vi "Postprocessing_utility_RA_molecularLine_fileSum.vi"() -> ()   [LabVIEW 2016]
doc: "VI for maser line post-processing"
uses:
  <vilib>/Utility/config.llb/Read Key (Double).vi
  <vilib>/Utility/file.llb/Read Delimited Spreadsheet (DBL).vi
  <vilib>/Utility/file.llb/Write Delimited Spreadsheet (DBL).vi
  <vilib>/Analysis/6fits.llb/1D B-Spline Fit.vi
  <vilib>/Utility/config.llb/NI_LVConfig.lvlib
  <vilib>/Analysis/NI_AALPro.lvlib
panel:
  in  "TabControl":enum32{"Averaging", "Jy&Speed plot"}(tab)
  in  "Frequency_MHz":dbl(knob)=969.0 caption="Frequency, MHz" min=70.0 max=6000.0 scale=70.0..6000.0 scale format="%#1_5g"
  out "Spectrum":cluster{dbl, dbl, dbl[]}(graph)={968.4, 0.0037406483790523685, [0.0, 0.0, 0.0, 0.0, 0.0, 0.0, 0.0, 0.0, 0.0, 0.0, 0.0, 0.0, 0.0, 0.0, 0.0, 0.0, 0.0, 0.0, 0.0, 0.0, 0.0, 0.0, 0.0, 0.0, 0.0, 0.0, 0.0, 0.0, 0.0, 0.0, 0.0, 0.0, 0.0, 0.0, 0.0, 0.0, 0.0, 0.0, 0.0, 0.0, 0.0, 0.0, 0.0, 0.0, 0.0, 0.0, 0.0, 0.0, 0.0, 0.0, 0.0, 0.0, 0.0, 0.0, 0.0, 0.0, 0.0, 0.0, 0.0, 0.0, 0.0, 0.0, 0.0, 0.0, 0.0, 0.0, 0.0, 0.0, 0.0, 0.0, 0.0, 0.0, 0.0, 0.0, 0.0, 0.0, 0.0, 0.0, 0.0, 0.0, 0.0, 0.0, 0.0, 0.0, 0.0, 0.0, 0.0, 0.0, 0.0, 0.0, 0.0, 0.0, 0.0, 0.0, 0.0, 0.0, 0.0, 0.0, 0.0, 0.0, 0.0, 0.0, 0.0, 0.0, 0.0, 0.0, 0.0, 0.0, 0.0, 0.0, 0.0, 0.0, 0.0, 0.0, 0.0, 0.0, 0.0, 0.0, 0.0, 0.0, 0.0, 0.0, 0.0, 0.0, 0.0, 0.0, 0.0, 0.0, 0.0, 0.0, 0.0, 0.0, 0.0, 0.0, 0.0, 0.0, 0.0, 0.0, 0.0, 0.0, 0.0, 0.0, 0.0, 0.0, 0.0, 0.0, 0.0, 0.0, 0.0, 0.0, 0.0, 0.0, 0.0, 0.0, 0.0, 0.0, 0.0, 0.0, 0.0, 0.0, 0.0, 0.0, 0.0, 0.0, 0.0, 0.0, 0.0, 0.0, 0.0, 0.0, 0.0, 0.0, 0.0, 0.0, 0.0, 0.0, 0.0, 0.0, 0.0, 0.0, 0.0, 0.0, 0.0, 0.0, 0.0, 0.0, 0.0, 0.0, 0.0, 0.0, 0.0, 0.0, 0.0, 0.0, 0.0, 0.0, 0.0, 0.0, 0.0, 0.0, 0.0, 0.0, 0.0, 0.0, 0.0, 0.0, 0.0, 0.0, 0.0, 0.0, 0.0, 0.0, 0.0, 0.0, 0.0, 0.0, 0.0, 0.0, 0.0, 0.0, 0.0, 0.0, 0.0, 0.0, 0.0, 0.0, 0.0, 0.0, 0.0, 0.0, 0.0, 0.0, 0.0, 0.0, 0.0, 0.0, 0.0, 0.0, 0.0, 0.0, 0.0, 0.0, 0.0, 0.0, 0.0, 0.0, 0.0, 0.0, 0.0, 0.0, 0.0, 0.0, 0.0, 0.0, 0.0, 0.0, 0.0, 0.0, 0.0, 0.0, 0.0, 0.0, 0.0, 0.0, 0.0, 0.0, 0.0, 0.0, 0.0, 0.0, 0.0, 0.0, 0.0, 0.0, 0.0, 0.0, 0.0, 0.0, 0.0, 0.0, 0.0, 0.0, 0.0, 0.0, 0.0, 0.0, 0.0, 0.0, 0.0, 0.0, 0.0, 0.0, 0.0, 0.0, 0.0, 0.0, 0.0, 0.0, 0.0, 0.0, 0.0, 0.0, 0.0, 0.0, 0.0, 0.0, 0.0, 0.0, 0.0, 0.0, 0.0, 0.0, 0.0, 0.0, 0.0, 0.0, 0.0, 0.0, 0.0, 0.0, 0.0, 0.0, 0.0, 0.0, 0.0, 0.0, 0.0, 0.0, 0.0, 0.0, 0.0, 0.0, 0.0, 0.0, 0.0, 0.0, 0.0, 0.0, 0.0, 0.0, 0.0, 0.0, 0.0, 0.0, 0.0, 0.0, 0.0, 0.0, 0.0, 0.0, 0.0, 0.0, 0.0, 0.0, 0.0, 0.0, 0.0, 0.0, 0.0, 0.0, 0.0, 0.0, 0.0, 0.0, 0.0, 0.0, 0.0, 0.0, 0.0, 0.0, 0.0, 0.0, 0.0, 0.0, 0.0, 0.0, 0.0, 0.0, 0.0, 0.0, 0.0, 0.0, 0.0, 0.0, 0.0, 0.0, 0.0, 0.0, 0.0, 0.0, 0.0, 0.0, 0.0, 0.0, 0.0, 0.0, 0.0, 0.0, 0.0, 0.0, 0.0]} caption="Power Spectrum"
  in  "FFT_size":dbl=333.0 caption="FFT size" min=128.0 max=28000000.0 step=1.0 format="%#_8g"
  out "Samplerate":dbl=1500000.0 caption="Sample rate (SR)" min=80000.0 max=40000000.0 step=1.0 format="%#_8g"
  in  "Bandwidth_MHz":dbl=1.5 caption="Bandwidth, MHz" min=1.5 max=28.0 format="%#_3g"
  in  "Plot_mult":dbl=1.0 caption="Plot mult" min=0.0 step=5.0
  in  "add_file":bool
  in  "stop":bool
  in  "Clear":bool
  out "last added":path
  in  "Fit":bool
  in  "Save":bool
  out "error":i32
  out "count":i32
  in  "points":dbl=25.0 format="%#_13g"
  in  "dB_scale":bool caption="dB/linear"
  in  "CFG name":string="USRP_line_monitor.cfg"
  in  "subtract_file":bool
  in  "bgr_mutl":dbl=1.0 caption="Alpha (back-gnd mult)" format="%#_13g"
  in  "subtract_reversed":bool
  in  "set_plot_ranges":bool
  in  "Jy_high":dbl=900.0 caption="Jy, high"
  in  "Jy_low":dbl=-200.0 caption="Jy, low"
  in  "VLSR_high":dbl=15.0 caption="VLSR high, km/s"
  in  "VLSR_low":dbl=-20.0 caption="VLSR low, km/s"
  in  "Vel_low":dbl=-40.87 caption="Velocity low, km/s"
  in  "Jy_vs_vel_plot":bool
  out "Spectrum_Jy_vel":cluster{dbl, dbl, dbl[]}(graph)={-40.87, 0.16817955112219451, [0.0, 0.0, 0.0, 0.0, 0.0, 0.0, 0.0, 0.0, 0.0, 0.0, 0.0, 0.0, 0.0, 0.0, 0.0, 0.0, 0.0, 0.0, 0.0, 0.0, 0.0, 0.0, 0.0, 0.0, 0.0, 0.0, 0.0, 0.0, 0.0, 0.0, 0.0, 0.0, 0.0, 0.0, 0.0, 0.0, 0.0, 0.0, 0.0, 0.0, 0.0, 0.0, 0.0, 0.0, 0.0, 0.0, 0.0, 0.0, 0.0, 0.0, 0.0, 0.0, 0.0, 0.0, 0.0, 0.0, 0.0, 0.0, 0.0, 0.0, 0.0, 0.0, 0.0, 0.0, 0.0, 0.0, 0.0, 0.0, 0.0, 0.0, 0.0, 0.0, 0.0, 0.0, 0.0, 0.0, 0.0, 0.0, 0.0, 0.0, 0.0, 0.0, 0.0, 0.0, 0.0, 0.0, 0.0, 0.0, 0.0, 0.0, 0.0, 0.0, 0.0, 0.0, 0.0, 0.0, 0.0, 0.0, 0.0, 0.0, 0.0, 0.0, 0.0, 0.0, 0.0, 0.0, 0.0, 0.0, 0.0, 0.0, 0.0, 0.0, 0.0, 0.0, 0.0, 0.0, 0.0, 0.0, 0.0, 0.0, 0.0, 0.0, 0.0, 0.0, 0.0, 0.0, 0.0, 0.0, 0.0, 0.0, 0.0, 0.0, 0.0, 0.0, 0.0, 0.0, 0.0, 0.0, 0.0, 0.0, 0.0, 0.0, 0.0, 0.0, 0.0, 0.0, 0.0, 0.0, 0.0, 0.0, 0.0, 0.0, 0.0, 0.0, 0.0, 0.0, 0.0, 0.0, 0.0, 0.0, 0.0, 0.0, 0.0, 0.0, 0.0, 0.0, 0.0, 0.0, 0.0, 0.0, 0.0, 0.0, 0.0, 0.0, 0.0, 0.0, 0.0, 0.0, 0.0, 0.0, 0.0, 0.0, 0.0, 0.0, 0.0, 0.0, 0.0, 0.0, 0.0, 0.0, 0.0, 0.0, 0.0, 0.0, 0.0, 0.0, 0.0, 0.0, 0.0, 0.0, 0.0, 0.0, 0.0, 0.0, 0.0, 0.0, 0.0, 0.0, 0.0, 0.0, 0.0, 0.0, 0.0, 0.0, 0.0, 0.0, 0.0, 0.0, 0.0, 0.0, 0.0, 0.0, 0.0, 0.0, 0.0, 0.0, 0.0, 0.0, 0.0, 0.0, 0.0, 0.0, 0.0, 0.0, 0.0, 0.0, 0.0, 0.0, 0.0, 0.0, 0.0, 0.0, 0.0, 0.0, 0.0, 0.0, 0.0, 0.0, 0.0, 0.0, 0.0, 0.0, 0.0, 0.0, 0.0, 0.0, 0.0, 0.0, 0.0, 0.0, 0.0, 0.0, 0.0, 0.0, 0.0, 0.0, 0.0, 0.0, 0.0, 0.0, 0.0, 0.0, 0.0, 0.0, 0.0, 0.0, 0.0, 0.0, 0.0, 0.0, 0.0, 0.0, 0.0, 0.0, 0.0, 0.0, 0.0, 0.0, 0.0, 0.0, 0.0, 0.0, 0.0, 0.0, 0.0, 0.0, 0.0, 0.0, 0.0, 0.0, 0.0, 0.0, 0.0, 0.0, 0.0, 0.0, 0.0, 0.0, 0.0, 0.0, 0.0, 0.0, 0.0, 0.0, 0.0, 0.0, 0.0, 0.0, 0.0, 0.0, 0.0, 0.0, 0.0, 0.0, 0.0, 0.0, 0.0, 0.0, 0.0, 0.0, 0.0, 0.0, 0.0, 0.0, 0.0, 0.0, 0.0, 0.0, 0.0, 0.0, 0.0, 0.0, 0.0, 0.0, 0.0, 0.0, 0.0, 0.0, 0.0, 0.0, 0.0, 0.0, 0.0, 0.0, 0.0, 0.0, 0.0, 0.0, 0.0, 0.0, 0.0, 0.0, 0.0, 0.0, 0.0, 0.0, 0.0, 0.0, 0.0, 0.0, 0.0, 0.0, 0.0, 0.0, 0.0, 0.0, 0.0, 0.0, 0.0, 0.0, 0.0, 0.0, 0.0, 0.0, 0.0, 0.0, 0.0, 0.0, 0.0, 0.0, 0.0, 0.0, 0.0, 0.0, 0.0, 0.0, 0.0, 0.0, 0.0, 0.0, 0.0]} caption="Power Spectrum"
  in  "Vel_high":dbl=26.57 caption="Velocity high, km/s"
  in  "Jy_mult":dbl=250000.0 caption="SEFD, Jy"
  in  "Jy_zero":dbl caption="Zero level adj., Jy"
  in  "Jy_slant_left":dbl caption="Slant corr. left, Jy"
  in  "Jy_slant_right":dbl caption="Slant corr. right, Jy"
  in  "Atm_atten_dB":dbl=0.2 caption="Atmospheric att., dB" min=0.0
  in  "line_high":dbl=-2.5 caption="Line high, km/s"
  in  "line_low":dbl=-5.0 caption="Line low, km/s"
  # "All files must be with equal number \nof the samples, averaging and other parameters"
  # "VLSRs corresponding to RX frequency band"
  # "Plot ranges"
  # "(applied after all \nadjustments and corrections)"
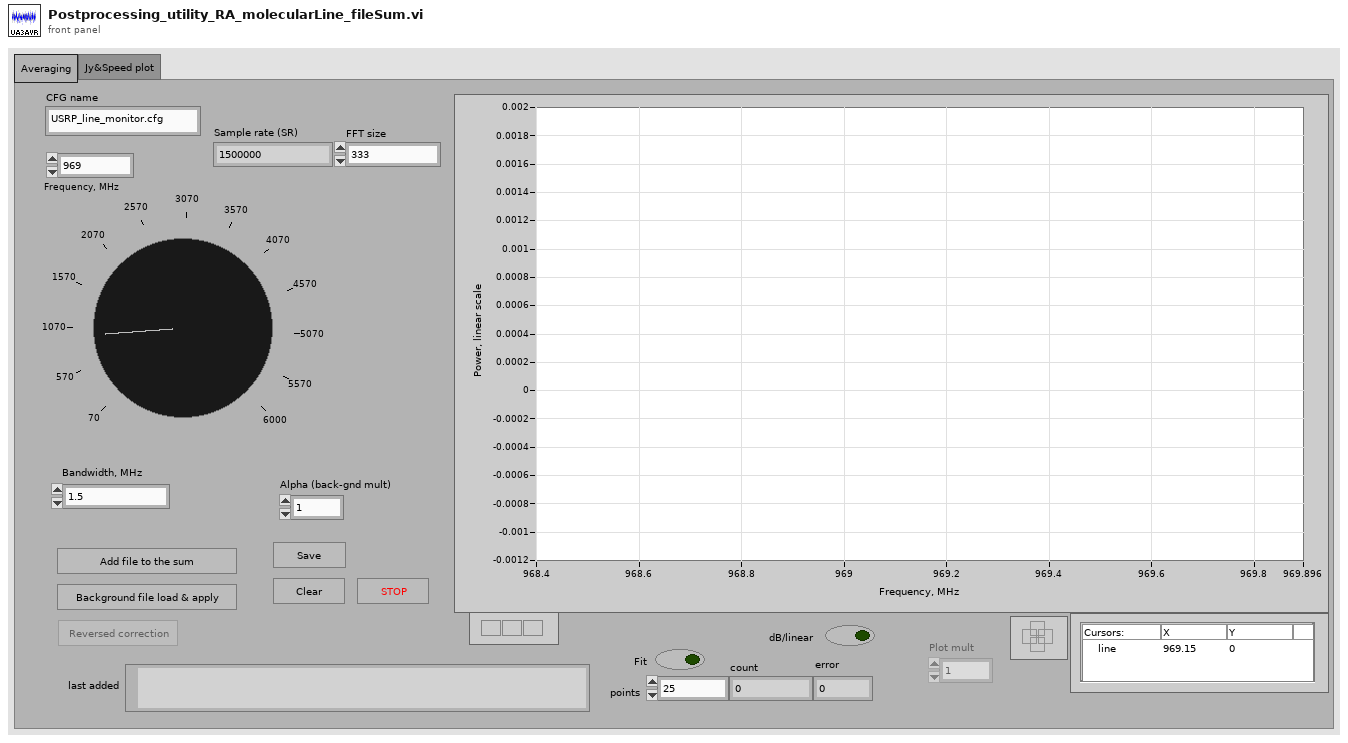
[diagram p1: front panel]
types:
  T1 = typedef "NI_LVConfig.lvlib/Config Data RefNum.ctl" = refnum<k1>
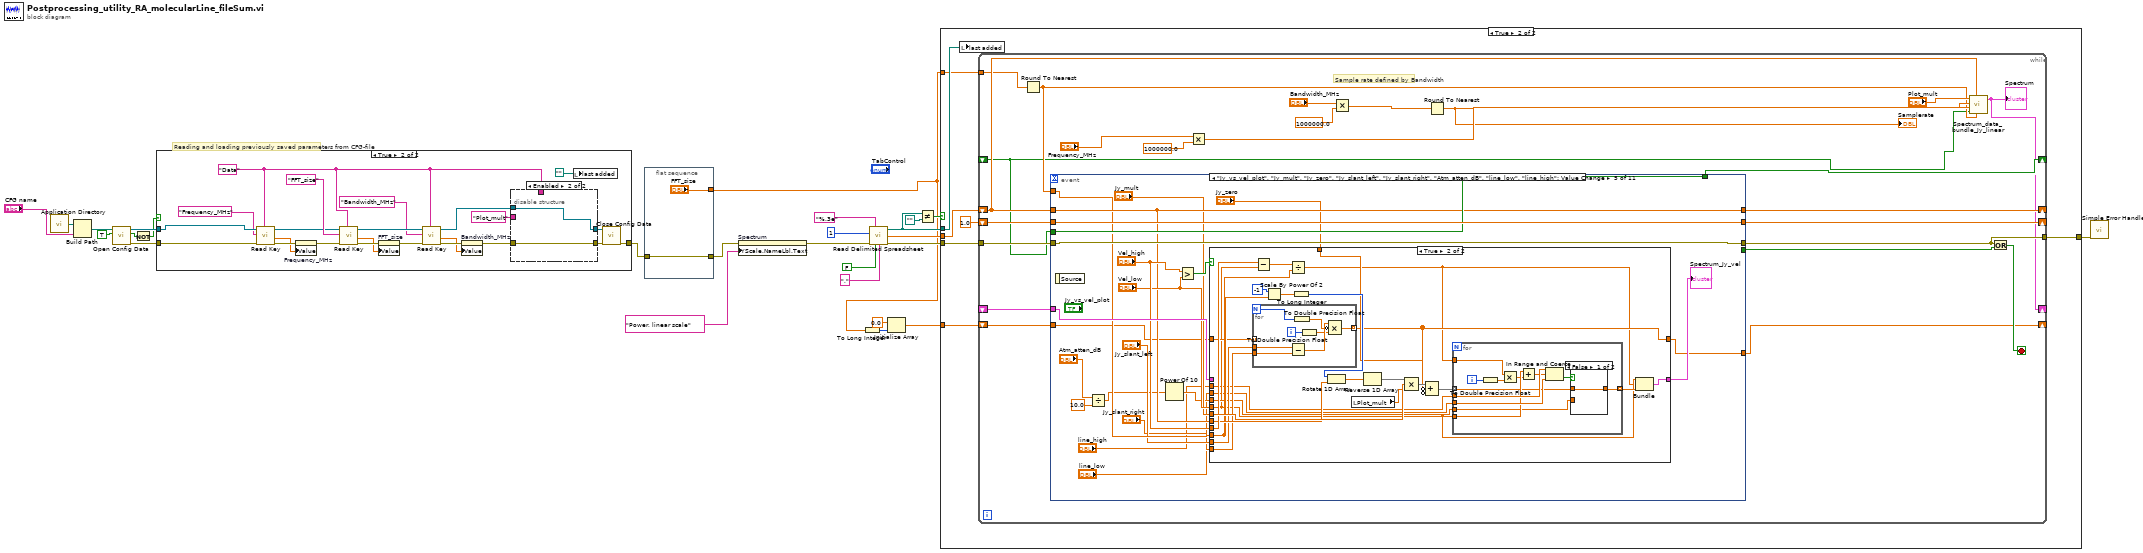
[diagram p0: block diagram]
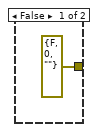
[diagram p2: hidden frame]
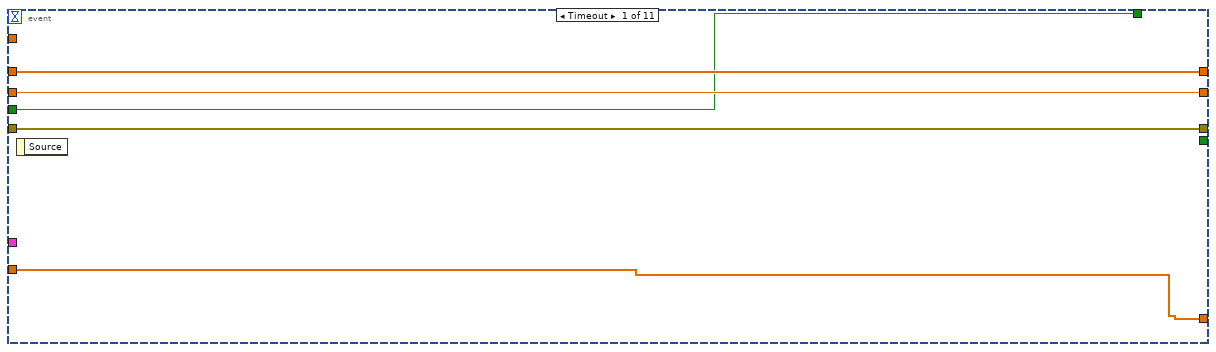
[diagram p3: hidden frame]
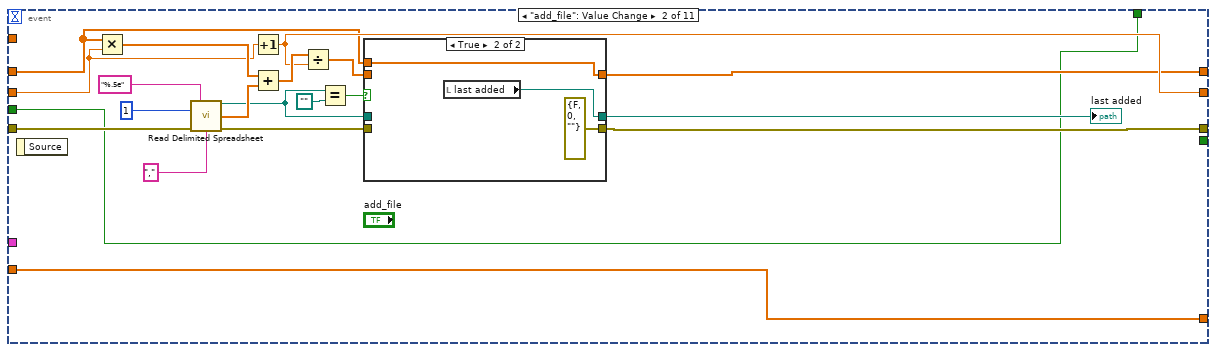
[diagram p4: hidden frame]
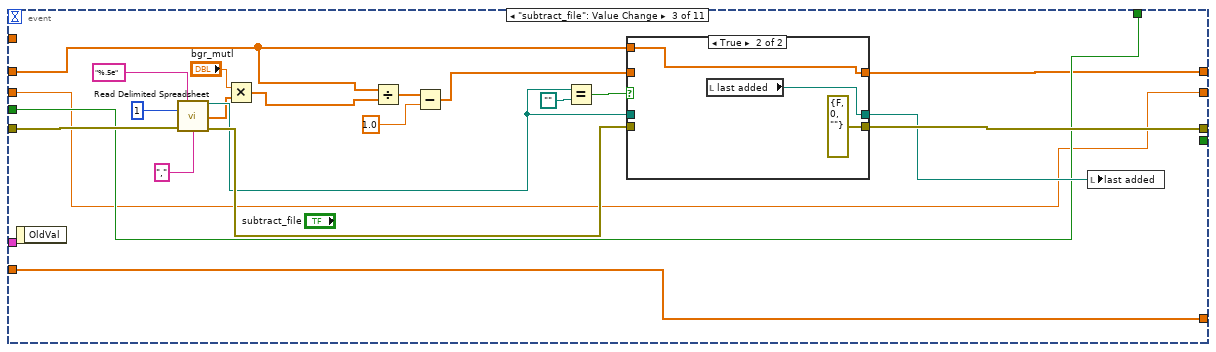
[diagram p6: hidden frame]
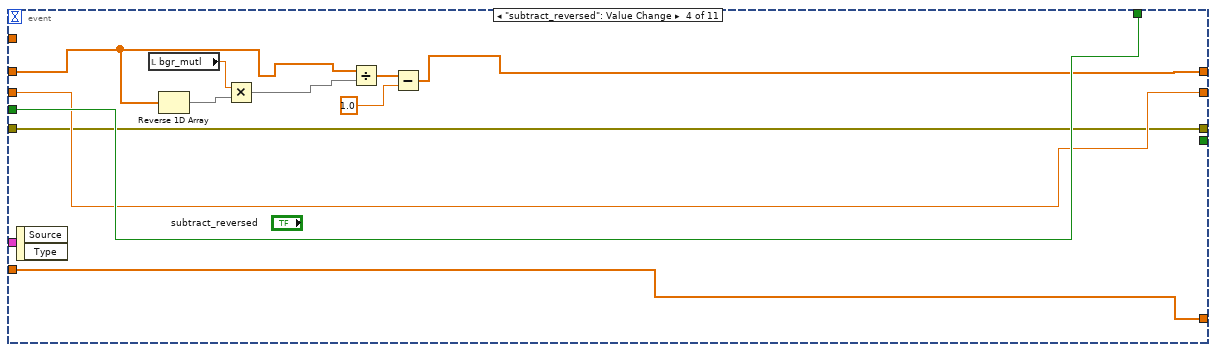
[diagram p8: hidden frame]
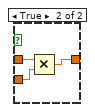
[diagram p10: hidden frame]
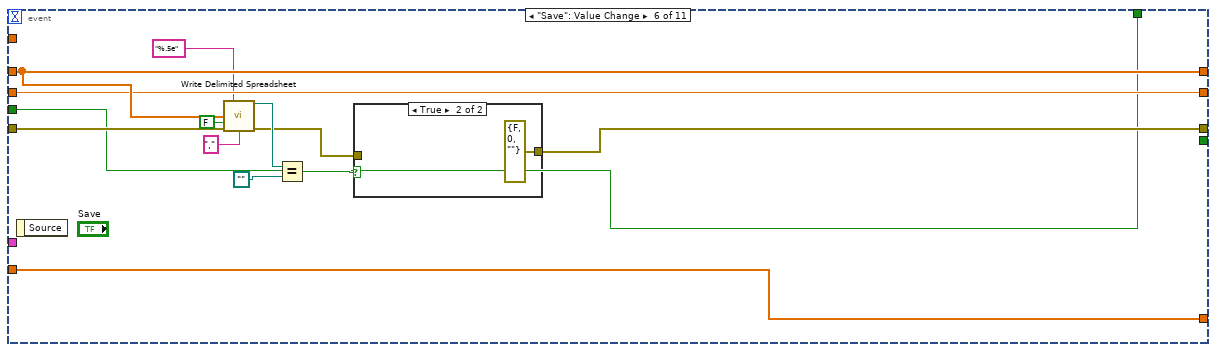
[diagram p11: hidden frame]
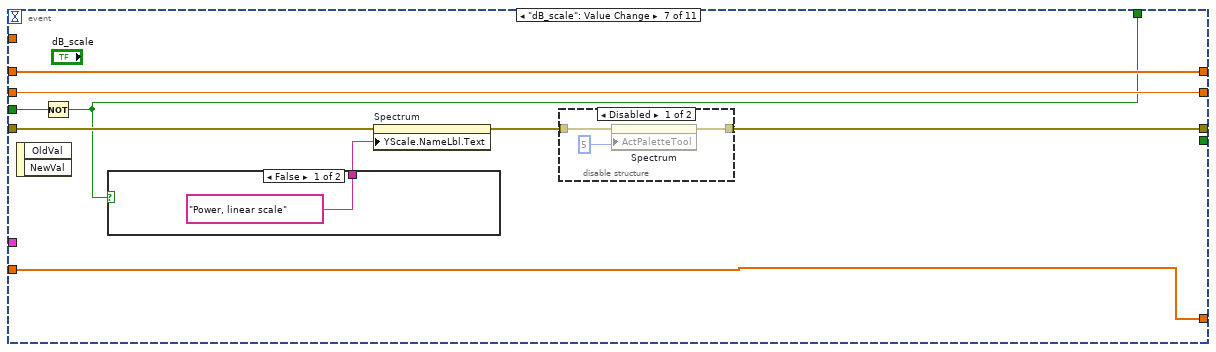
[diagram p13: hidden frame]
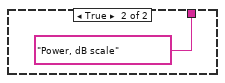
[diagram p15: hidden frame]
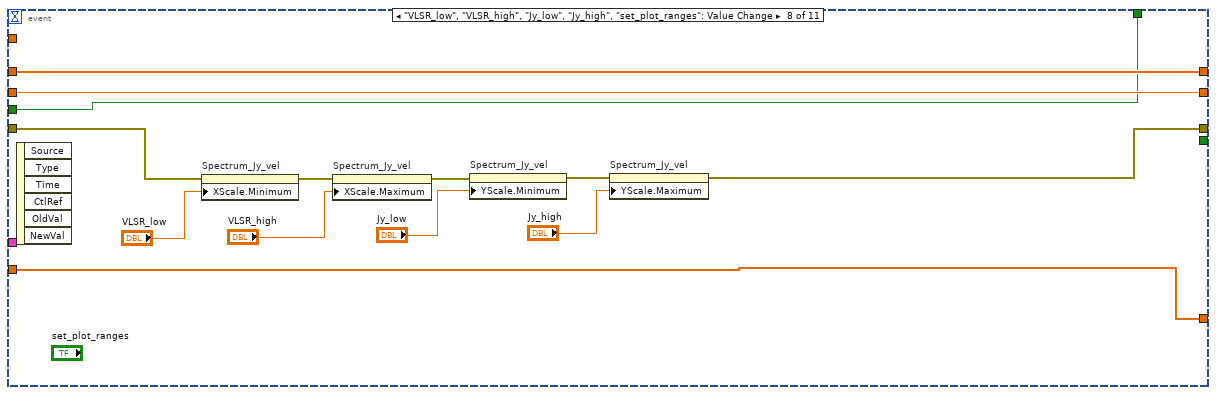
[diagram p16: hidden frame]
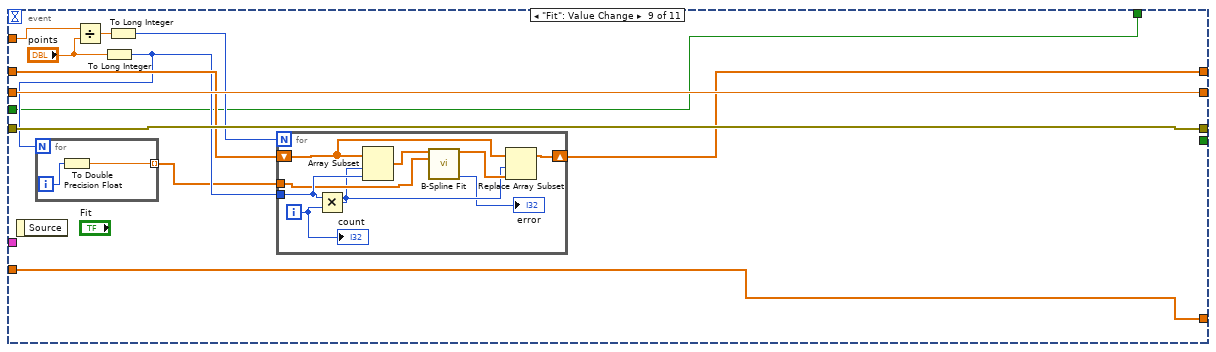
[diagram p17: hidden frame]
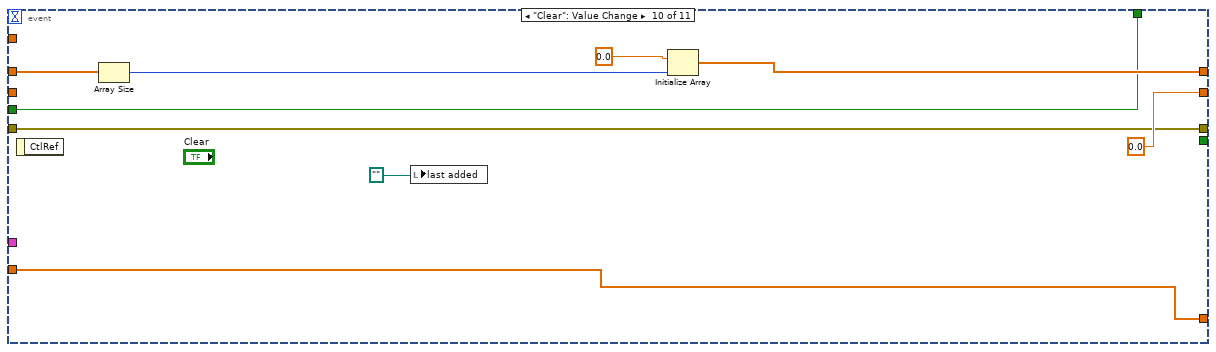
[diagram p18: hidden frame]
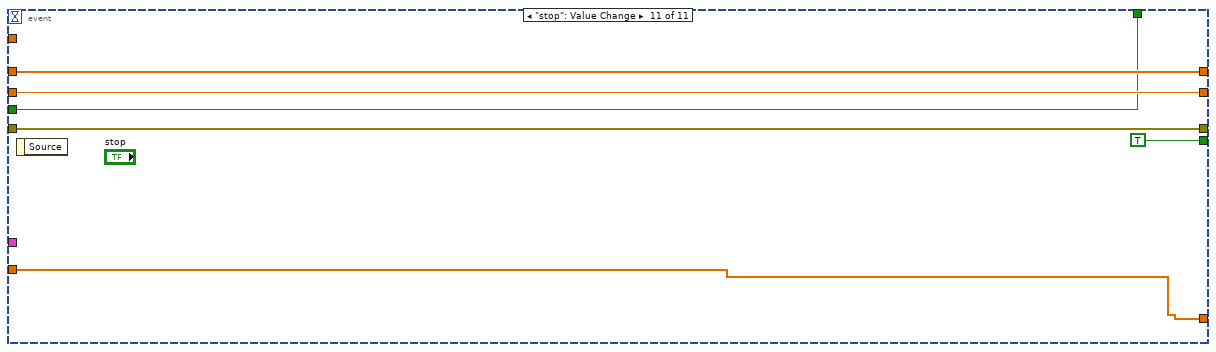
[diagram p19: hidden frame]
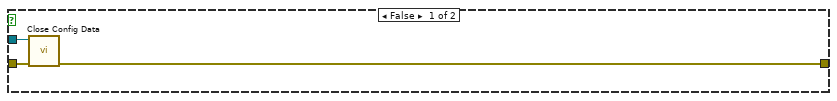
[diagram p20: hidden frame]
diagram:
  # "Reading and loading previously saved parameters from CFG-file"
  n1 = call <vilib>:"Application Directory.vi"() -> ("Application Directory"=w13:path)
  n2 = Build Path(base path=w13, name or relative path="CFG name") -> (appended path=w19:path)
  n3 = call <vilib>:"Open Config Data.vi"("create file if necessary (T)"=TRUE, "configuration file path"=w19) -> ("error out"=w17:errorcluster, "file created?"=w15:bool, "refnum"=w18:T1)  [unwired: 7 in]
  n4 = Not(x=w15) -> (.not. x?=w14:bool)
  n5 = case shown="True" w14 {
    tunnel: w18 -> [w27 w52]
    tunnel: w17 -> [w29 w51]
    tunnel: [w28 w50] -> w3
    frame False {
      n6 = call <vilib>:"Close Config Data.vi"("error in (no error)"=w29, "refnum"=w27) -> ("error out"=w28:errorcluster)  [unwired: 8 in, 1 out]
    }
    frame True {
      w37 = "Data" ("section")
      n7 = call-poly <vilib>:"Read Key.vi"("section"=w37, "error in (no error)"=w51, "key"="Frequency_MHz", "refnum"=w52) -> ("error out"=w36:errorcluster, "value"=w32:dbl, "refnum out"=w35:T1)  [unwired: 4 in, 1 out]
      n8 = property on="Frequency_MHz" class="Knob (strict)"(error in=w36, "Value"=w32) -> (error out=w47:errorcluster)  [unwired: 1 in, 1 out]
      n9 = call-poly <vilib>:"Read Key.vi"("section"=w37, "error in (no error)"=w47, "key"="FFT_size" ("Control Name"), "refnum"=w35) -> ("error out"=w49:errorcluster, "value"=w48:dbl, "refnum out"=w42:T1)  [unwired: 4 in, 1 out]
      n10 = property on="FFT_size" class="DigNum (strict)"(error in=w49, "Value"=w48) -> (error out=w43:errorcluster)  [unwired: 1 in, 1 out]
      n11 = call-poly <vilib>:"Read Key.vi"("section"=w37, "error in (no error)"=w43, "key"="Bandwidth_MHz" ("Control Name"), "refnum"=w42) -> ("error out"=w45:errorcluster, "value"=w44:dbl, "refnum out"=w39:T1)  [unwired: 4 in, 1 out]
      n12 = property on="Bandwidth_MHz" class="DigNum (strict)"(error in=w45, "Value"=w44) -> (error out=w40:errorcluster)  [unwired: 1 in, 1 out]
      n13 = disable-structure shown="Enabled" {
        disable-tunnel: w40 -> [w58 w61]
        disable-tunnel: w39 -> [w57 w60]
        disable-tunnel: "Plot_mult" ("Control Name") -> [w56 _]
        disable-tunnel: w37 -> [w55 _]
        disable-tunnel: [w54 w61] -> w34
        disable-tunnel: [w53 w60] -> w33
        frame Disabled {
          n14 = call-poly <vilib>:"Read Key.vi"("section"=w55, "error in (no error)"=w58, "key"=w56, "refnum"=w57) -> ("error out"=w59:errorcluster, "refnum out"=w53:T1)  [unwired: 4 in, 2 out]
          n15 = property on="Plot_mult" class="DigNum (strict)" props=["Value"](error in=w59) -> (error out=w54:errorcluster)  [unwired: 2 in, 1 out]
        }
        frame Enabled {
        }
      }
      n16 = local write "last added"(path "") -> ()
      n17 = call <vilib>:"Close Config Data.vi"("error in (no error)"=w34, "refnum"=w33) -> ("error out"=w50:errorcluster)  [unwired: 8 in, 1 out]
    }
  }
  n18 = flat-sequence {
    tunnel: w3 -> [w63]
    tunnel: [w63] -> w2
    tunnel: ["FFT_size"] -> w1
    frame #0 {
    }
  }
  n19 = property on="Spectrum" class="WFGraph (strict)"(error in=w2, "YScale.NameLbl.Text"="Power, linear scale") -> (error out=w8:errorcluster)  [unwired: 1 in, 1 out]
  n20 = To Long Integer(number=w1) -> (32bit integer=w5:i32)
  n21 = call-poly <vilib>:"Read Delimited Spreadsheet.vi"("format (%.3f)"="%.3e", "number of rows (all:-1)"=1, "error in (no error)"=w8, "transpose? (F)"=FALSE, "delimiter (\\t)"="," ("delimiter (\\t)")) -> ("new file path (Not A Path if cancelled)"=w9:path, "first row"=w24:dbl[], "error out"=w21:errorcluster)  [unwired: 5 in, 3 out]
  n22 = Initialize Array(0.0 ("element"), w5) -> (w4:dbl[])
  n23 = Not Equal?(x=w9, y=path "") -> (x != y?=w10:bool)
  n24 = case shown="True" w10 {
    tunnel: w24 -> [_ w71]
    tunnel: w21 -> [_ w70]
    tunnel: [errorcluster {"status"=FALSE, "code"=0, "source"=""} ("error out") w68] -> w12
    tunnel: w9 -> [_ w67]
    tunnel: w1 -> [_ w66]
    tunnel: w4 -> [_ w65]
    frame False {
    }
    frame True {
      n25 = local write "last added"(w67) -> ()
      n26 = while {
        shift-right: [w82] -> _
        shift-left: w71 -> [w81]
        tunnel: w70 -> [w88]
        tunnel: [w87] -> w68
        shift-right: [w83] -> _
        shift-left: 1.0 -> [w84]
        shift-right: [w79] -> _
        shift-left: _ -> [w78]
        shift-right: [w77] -> _
        shift-left: _ -> [w76]
        tunnel: w66 -> [w75]
        shift-right: [w73] -> _
        shift-left: w65 -> [w74]
        stop <- w85 stop-if-true
        # "Sample rate defined by Bandwidth"
        n27 = Round To Nearest(number=w75) -> (nearest integer value=w80:dbl)
        n28 = event shown="[4] \"Jy_vs_vel_plot\", \"Jy_mult\", \"Jy_zero\", \"Jy_slant_left\", \"Jy_slant_right\", \"Atm_atten_dB\", \"line_low\", \"line_high\": Value Change" {
          selector: _ -> [_ _ _ _ _ _ _ _ _ _ _]
          dyn-events: _ -> [_ _ _ _ _ _ _ _ _ _ _]
          timeout: _ -> [_ _ _ _ _ _ _ _ _ _ _]
          tunnel: w81 -> [w99 w109 w132 w157 w178 w250 w260 w279 w287 w311 w318]
          tunnel: w88 -> [w100 w118 w139 w161 w184 w248 w258 w270 w291 w307 w317]
          tunnel: [w100 w103 w138 w161 w184 w240 w254 w271 w291 w307 w317] -> w87
          tunnel: [w99 w107 w135 w156 w178 w250 w260 w279 w283 w308 w318] -> w82
          tunnel: [_ _ _ _ _ _ _ _ _ _ TRUE] -> w86
          tunnel: [w98 w112 w134 w163 w186 w249 w261 w280 w292 0.0 w315] -> w83
          tunnel: w84 -> [w98 w114 w134 w163 w186 w249 w261 w280 w292 _ w315]
          tunnel: w80 -> [_ _ _ _ w175 _ _ _ w289 _ _]
          tunnel: [w97 w102 w136 w164 w185 w239 w257 w277 w282 w305 w314] -> w79
          tunnel: w78 -> [w97 w102 w136 w164 w185 w239 w259 w277 w282 w305 w314]
          tunnel: w76 -> [_ _ _ _ w181 _ _ _ _ _ _]
          tunnel: w74 -> [w96 w101 w129 w159 w174 w238 w253 w278 w281 w304 w313]
          tunnel: [w96 w101 w129 w159 w171 w238 w253 w278 w281 w304 w313] -> w73
          event Timeout {
            n29 = event-data() -> ()  [unwired: 1 in, 1 out]
          }
          event "add_file": Value Change {
            n30 = event-data() -> ()  [unwired: 1 in, 1 out]
            n31 = Multiply(x=w109, y=w114) -> (x*y=w115:dbl[])
            n32 = call-poly <vilib>:"Read Delimited Spreadsheet.vi"("format (%.3f)"="%.5e", "number of rows (all:-1)"=1, "error in (no error)"=w118, "delimiter (\\t)"="," ("delimiter (\\t)")) -> ("new file path (Not A Path if cancelled)"=w106:path, "first row"=w116:dbl[], "error out"=w104:errorcluster)  [unwired: 6 in, 3 out]
            n33 = Increment(x=w114) -> (x+1=w112:dbl)
            n34 = Add(x=w115, y=w116) -> (x+y=w113:dbl[])
            n35 = Divide(x=w113, y=w112) -> (x/y=w108:dbl[])
            n36 = Equal?(x=w106, y=path "") -> (x = y?=w110:bool)
            n37 = case shown="True" w110 {
              tunnel: w109 -> [_ w126]
              tunnel: w108 -> [w123 _]
              tunnel: [w123 w126] -> w107
              tunnel: w106 -> [w122 _]
              tunnel: [w122 w124] -> w105
              tunnel: w104 -> [w121 _]
              tunnel: [w121 errorcluster {"status"=FALSE, "code"=0, "source"=""} ("error out")] -> w103
              frame False {
              }
              frame True {
                n38 = local read "last added"() -> (w124:path)
              }
            }
            "last added" <- w105
          }
          event "subtract_file": Value Change {
            n39 = event-data() -> ()  [unwired: 1 in, 1 out]
            n40 = call-poly <vilib>:"Read Delimited Spreadsheet.vi"("format (%.3f)"="%.5e", "number of rows (all:-1)"=1, "error in (no error)"=w139, "delimiter (\\t)"="," ("delimiter (\\t)")) -> ("new file path (Not A Path if cancelled)"=w146:path, "first row"=w143:dbl[], "error out"=w147:errorcluster)  [unwired: 6 in, 3 out]
            n41 = Multiply(x="bgr_mutl", y=w143) -> (x*y=w131:dbl[])
            n42 = Divide(x=w132, y=w131) -> (x/y=w128:dbl[])
            n43 = Subtract(x=w128, y=1.0) -> (x-y=w133:dbl[])
            n44 = Equal?(x=w146, y=path "") -> (x = y?=w145:bool)
            n45 = case shown="True" w145 {
              tunnel: w133 -> [w150 _]
              tunnel: [w150 w151] -> w135
              tunnel: w146 -> [w149 _]
              tunnel: [w149 w152] -> w137
              tunnel: w147 -> [w148 _]
              tunnel: [w148 errorcluster {"status"=FALSE, "code"=0, "source"=""} ("error out")] -> w138
              tunnel: w132 -> [_ w151]
              frame False {
              }
              frame True {
                n46 = local read "last added"() -> (w152:path)
              }
            }
            n47 = local write "last added"(w137) -> ()
          }
          event "subtract_reversed": Value Change {
            n48 = event-data() -> ()  [unwired: 1 in, 2 out]
            n49 = local read "bgr_mutl"() -> (w162:dbl)
            n50 = Reverse 1D Array(array=w157) -> (reversed array=w160:dbl[])
            n51 = Multiply(x=w162, y=w160) -> (x*y=w158:dbl[])
            n52 = Divide(x=w157, y=w158) -> (x/y=w155:dbl[])
            n53 = Subtract(x=w155, y=1.0) -> (x-y=w156:dbl[])
          }
          event "Jy_vs_vel_plot", "Jy_mult", "Jy_zero", "Jy_slant_left", "Jy_slant_right", "Atm_atten_dB", "line_low", "line_high": Value Change {
            n54 = event-data() -> ()  [unwired: 1 in, 1 out]
            n55 = Divide(x="Atm_atten_dB", y=10.0) -> (x/y=w167:dbl)
            n56 = Power Of 10(x=w167) -> (10^x=w168:dbl)
            n57 = Greater?(x="Vel_high", y="Vel_low") -> (0:w183:bool)
            n58 = case shown="True" w183 {
              tunnel: [w188 w193] -> w182
              tunnel: w181 -> [w188 _]
              tunnel: "Vel_high" -> [_ w210]
              tunnel: "Vel_low" -> [_ w192]
              tunnel: w175 -> [_ w201]
              tunnel: w178 -> [_ w206]
              tunnel: "Jy_mult" -> [_ w212]
              tunnel: "Jy_zero" -> [_ w202]
              tunnel: w174 -> [w187 w200]
              tunnel: "Jy_slant_left" -> [_ w199]
              tunnel: "Jy_slant_right" -> [_ w198]
              tunnel: [w187 w197] -> w171
              tunnel: w168 -> [_ w195]
              tunnel: "line_high" -> [_ w191]
              tunnel: "line_low" -> [_ w190]
              frame False {
              }
              frame True {
                n59 = for {
                  N -> [w234]
                  tunnel: w200 -> [_] mode=indexing
                  tunnel: w199 -> [w236]
                  tunnel: w198 -> [w235]
                  tunnel: [w232] -> w197 mode=indexing
                  i -> [w231]
                  n60 = Subtract(x=w236, y=w235) -> (x-y=w237:dbl)
                  n61 = To Double Precision Float(number=w234) -> (double precision float=w233:dbl)
                  n62 = To Double Precision Float(number=w231) -> (double precision float=w230:dbl)
                  n63 = Compound Arithmetic op=MULTIPLY(w237, invert w233, w230) -> (w232:dbl)
                }
                n64 = Subtract(x=w210, y=w192) -> (x-y=w213:dbl)
                n65 = Scale By Power Of 2(n=i16 -1, x=w201) -> (x*2^n=w208:dbl)
                n66 = Divide(x=w213, y=w201) -> (x/y=w189:dbl)
                n67 = To Long Integer(number=w208) -> (32bit integer=w207:i32)
                n68 = Rotate 1D Array(1:w206, 2:w207) -> (0:w211:dbl[])
                n69 = local read "Plot_mult"() -> (w205:dbl)
                n70 = Reverse 1D Array(array=w211) -> (reversed array=w204:dbl[])
                n71 = Compound Arithmetic op=MULTIPLY(w204, w212, w205) -> (w203:dbl[])
                n72 = Compound Arithmetic op=ADD(w203, invert w202, invert w197) -> (w196:dbl[])
                n73 = for {
                  tunnel: w196 -> [w215] mode=indexing
                  tunnel: w195 -> [w214]
                  tunnel: [w225] -> w194 mode=indexing
                  tunnel: w192 -> [w221]
                  tunnel: w191 -> [w224]
                  tunnel: w190 -> [w223]
                  tunnel: w189 -> [w218]
                  i -> [w220]
                  n74 = To Double Precision Float(number=w220) -> (double precision float=w217:dbl)
                  n75 = Multiply(x=w218, y=w217) -> (x*y=w219:dbl)
                  n76 = Add(x=w221, y=w219) -> (x+y=w222:dbl)
                  n77 = In Range and Coerce(upper limit=w224, x=w222, lower limit=w223) -> (In Range?=w216:bool)  [unwired: 1 out]
                  n78 = case shown="False" w216 {
                    tunnel: [w226 w229] -> w225
                    tunnel: w215 -> [w226 w228]
                    tunnel: w214 -> [_ w227]
                    frame False {
                    }
                    frame True {
                      n79 = Multiply(x=w228, y=w227) -> (x*y=w229:dbl)
                    }
                  }
                }
                n80 = Bundle("Vel_low"=w192, w189, w194) -> (w193:cluster{"Vel_low":dbl, dbl, dbl[]})  [unwired: 1 in]
              }
            }
            "Spectrum_Jy_vel" <- w182
          }
          event "Save": Value Change {
            n81 = event-data() -> ()  [unwired: 1 in, 1 out]
            n82 = call-poly <vilib>:"Write Delimited Spreadsheet.vi"("format (%.3f)"="%.5e", "1D data"=w250, "append to file? (new file:F)"=FALSE, "error in (no error)"=w248, "delimiter (\\t)"="," ("delimiter (\\t)")) -> ("new file path (Not A Path if cancelled)"=w244:path, "error out"=w241:errorcluster)  [unwired: 9 in]
            n83 = Equal?(x=w244, y=path "") -> (x = y?=w242:bool)
            n84 = case shown="True" w242 {
              tunnel: w241 -> [w251 _]
              tunnel: [w251 errorcluster {"status"=FALSE, "code"=0, "source"=""} ("error out")] -> w240
              frame False {
              }
              frame True {
              }
            }
          }
          event "dB_scale": Value Change {
            n85 = event-data() -> ()  [unwired: 1 in, 2 out]
            n86 = Not(x=w259) -> (.not. x?=w257:bool)
            n87 = case shown="False" w257 {
              tunnel: ["Power, linear scale" "Power, dB scale"] -> w256
              frame False {
              }
              frame True {
              }
            }
            n88 = property on="Spectrum" class="WFGraph (strict)"(error in=w258, "YScale.NameLbl.Text"=w256) -> (error out=w255:errorcluster)  [unwired: 1 in, 1 out]
            n89 = disable-structure shown="Disabled" {
              disable-tunnel: w255 -> [w264 w265]
              disable-tunnel: [w263 w265] -> w254
              frame Disabled {
                n90 = property on="Spectrum" class="WFGraph (strict)"(error in=w264, "ActPaletteTool"=5 ("Palette:Active Tool")) -> (error out=w263:errorcluster)  [unwired: 1 in, 1 out]
              }
              frame Enabled {
              }
            }
          }
          event "VLSR_low", "VLSR_high", "Jy_low", "Jy_high", "set_plot_ranges": Value Change {
            n91 = event-data() -> ()  [unwired: 1 in, 6 out]
            n92 = property on="Spectrum_Jy_vel" class="WFGraph (strict)"(error in=w270, "XScale.Minimum"="VLSR_low") -> (error out=w276:errorcluster)  [unwired: 1 in, 1 out]
            n93 = property on="Spectrum_Jy_vel" class="WFGraph (strict)"(error in=w276, "XScale.Maximum"="VLSR_high") -> (error out=w273:errorcluster)  [unwired: 1 in, 1 out]
            n94 = property on="Spectrum_Jy_vel" class="WFGraph (strict)"(error in=w273, "YScale.Minimum"="Jy_low") -> (error out=w272:errorcluster)  [unwired: 1 in, 1 out]
            n95 = property on="Spectrum_Jy_vel" class="WFGraph (strict)"(error in=w272, "YScale.Maximum"="Jy_high") -> (error out=w271:errorcluster)  [unwired: 1 in, 1 out]
          }
          event "Fit": Value Change {
            n96 = event-data() -> ()  [unwired: 1 in, 1 out]
            n97 = Divide(x=w289, y="points") -> (x/y=w290:dbl)
            n98 = To Long Integer(number="points") -> (32bit integer=w285:i32)
            n99 = for {
              N: w285 -> [_]
              tunnel: [w293] -> w284 mode=indexing
              i -> [w294]
              n100 = To Double Precision Float(number=w294) -> (double precision float=w293:dbl)
            }
            n101 = To Long Integer(number=w290) -> (32bit integer=w288:i32)
            n102 = for {
              N: w288 -> [_]
              tunnel: w285 -> [w302]
              tunnel: w284 -> [w300]
              shift-right: [w299] -> w283
              shift-left: w287 -> [w298]
              i -> [w303]
              n103 = Multiply(x=w302, y=w303) -> (x*y=w296:i32)
              n104 = Array Subset(array=w298, index=w296, length=w302) -> (w301:dbl[])
              n105 = call-poly <vilib>:"B-Spline Fit.vi"("Y"=w301, "X"=w300) -> ("Best BSpline Fit Y"=w297:dbl[], "error"=→"error":i32)  [unwired: 10 in, 2 out]
              n106 = Replace Array Subset(array=w298, new element=w297, index=w296) -> (w299:dbl[])
              "count" <- w303
            }
          }
          event "Clear": Value Change {
            n107 = event-data() -> ()  [unwired: 1 in, 1 out]
            n108 = Array Size(array=w311) -> (size(s)=w310:i32)
            n109 = local write "last added"(path "") -> ()
            n110 = Initialize Array(0.0 ("element"), w310) -> (w308:dbl[])
          }
          event "stop": Value Change {
            n111 = event-data() -> ()  [unwired: 1 in, 1 out]
          }
        }
        n112 = Multiply(x="Frequency_MHz", y=1000000.0) -> (x*y=w91:dbl)
        n113 = Multiply(x="Bandwidth_MHz", y=1000000.0) -> (x*y=w72:dbl)
        n114 = Round To Nearest(number=w72) -> (nearest integer value=w90:dbl)
        "Samplerate" <- w90
        n115 = call "Spectrum_data_bundle_Jy_linear.vi"("FFT size"=w80, "Power spectrum input"=w81, "dB_scale"=w78, "Central frequency, Hz"=w91, "Sample Rate"=w90, "Plot mult"="Plot_mult") -> ("Output cluster to waveform graph"=w77:cluster{dbl, dbl, dbl[]})  [unwired: 5 in]
        "Spectrum" <- w77
        n116 = Or(x=w87, y=w86) -> (x .or. y?=w85:bool)
      }
    }
  }
  n117 = call <vilib>:"Simple Error Handler.vi"("error in (no error)"=w12) -> ()  [unwired: 4 in, 5 out]
